vi "QR_code_Check_St1.vi"(5 "Columns":string[](array[string]), 7 "error in (no error)":errorcluster, 8 "replace %s":string, 9 "table":string, 10 "Refnum in":T1) -> (0 "error out":errorcluster, 1 "data":string[][](array[string]), 2 "TRUE no barcode Done on station 1":bool, 3 "Refnum out":T1, 4 "resulting string":string)   [LabVIEW 2017]
uses:
  <vilib>/addons/database/Connection.llb/Conn ObjectReference.ctl
  <vilib>/addons/database/NI_Database_API.lvlib
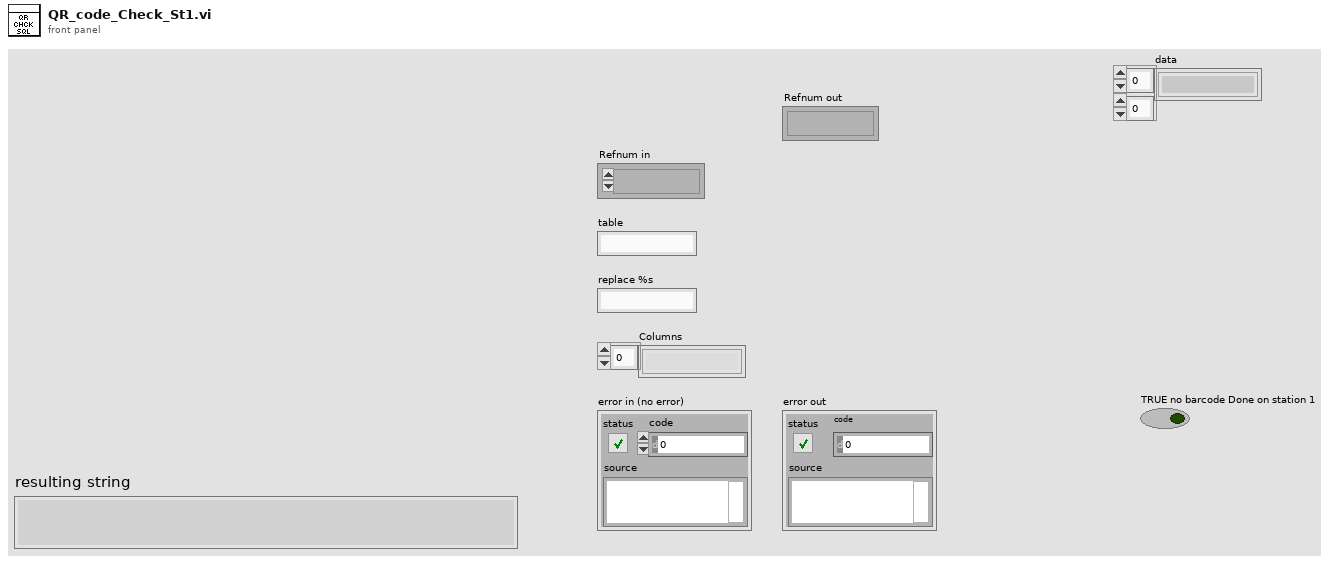
[diagram p1: front panel]
types:
  T1 = typedef "NI_Database_API.lvlib/Conn ObjectReference.ctl" = refnum<k1>
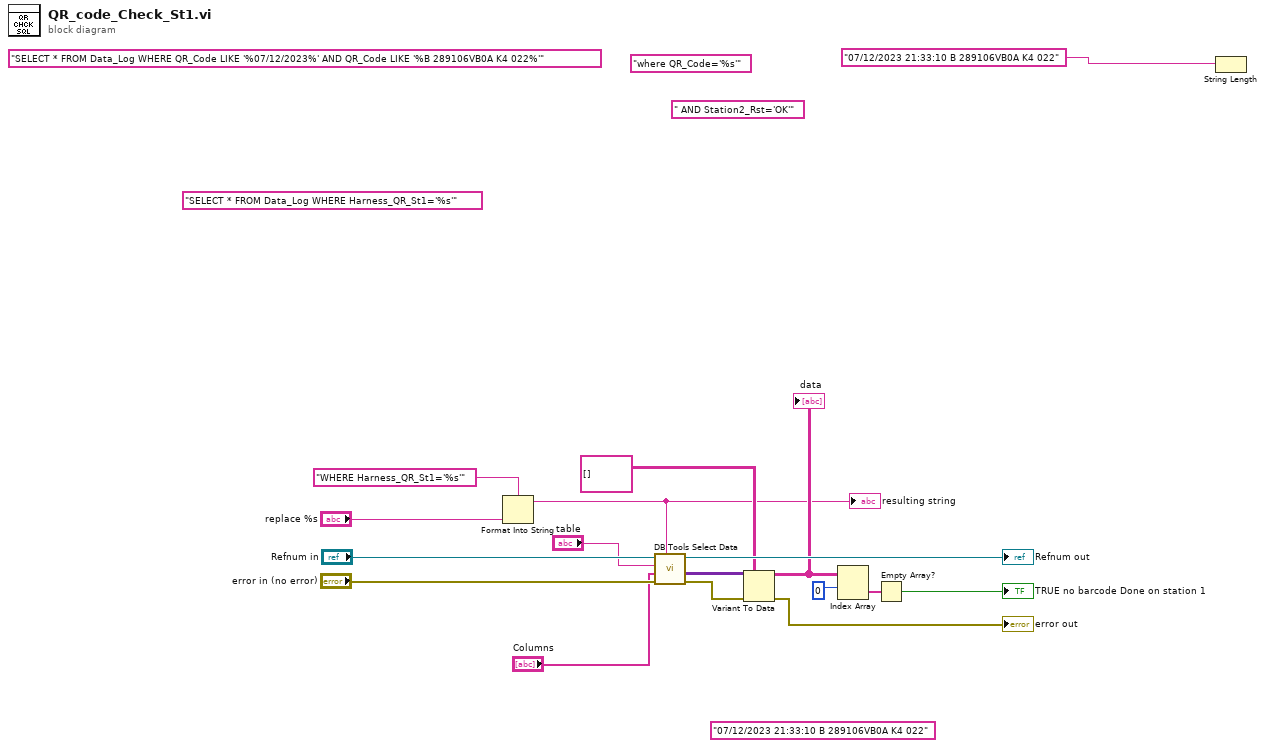
[diagram p0: block diagram]
diagram:
  (unwired) "SELECT * FROM Data_Log WHERE Harness_QR_St1='%s'" ("format string")
  (unwired) "07/12/2023 21:33:10 B 289106VB0A K4 022" ("format string")
  (unwired) "SELECT * FROM Data_Log WHERE QR_Code LIKE '%07/12/2023%' AND QR_Code LIKE '%B 289106VB0A K4 022%'" ("format string")
  (unwired) "where QR_Code='%s'" ("format string")
  (unwired) " AND Station2_Rst='OK'" ("replace %s")
  n1 = Format Into String(format string="WHERE Harness_QR_St1='%s'", "replace %s") -> (resulting string=w3:string)  [unwired: 2 in, 1 out]
  "resulting string" <- w3
  n2 = call <vilib>:"DB Tools Select Data.vi"("condition"=w3, "error in (no error)"="error in (no error)", "columns"="Columns", "table"="table", "connection reference"="Refnum in") -> ("error out"=w8:errorcluster, "data"=w10:variant[][], "connection reference out"=→"Refnum out":T1)  [unwired: 1 in]
  n3 = Variant To Data(error in=w8, type=string[][] [], Variant=w10) -> (data=w9:string[][], error out=→"error out":errorcluster)
  "data" <- w9
  n4 = Index Array(array=w9, index (row)=0) -> (element=w7:string[])  [unwired: 1 in]
  n5 = Empty Array?(array=w7) -> (empty?=→"TRUE no barcode Done on station 1":bool)
  n6 = String Length(string="07/12/2023 21:33:10 B 289106VB0A K4 022" ("format string")) -> ()  [unwired: 1 out]
